vi "TEST_TankControl.vi"() -> ()   [LabVIEW 2024]
doc: "This example performs writes and reads on a serial port, as directed by the user. You can press the Write and Read buttons, and change the Read Count, while the example is running.\n\nThe parameters set for the serial port must match the parameters of the connected instrument or device. In this example, the Read Count parameter specifies the number of bytes that the serial port reads. If there were more bytes at the port than the specified number, those bytes would not be read. If there were less bytes at the port than the specified number, you would receive a timeout error.\n\nThis example expands upon the flow control options for XON and XOFF, allowing the user to choose those control characters. Also, the user can enable or disable a termination character. Some devices require a termination character in order to identify the end of command strings. Some devices send a termination character to signify the end of data to be read. This example shows how you can end the Read operation once a termination character is detected in the buffer and/or append a termination character at the end of the Write data."
uses:
  LabVIEW_InstrDriver_forLK-G3000_ver1_0_1_0/32bit/Keyence LK-G3000/Public/clusters/LKIF_FLOATVALUE.ctl
  LabVIEW_InstrDriver_forLK-G3000_ver1_0_1_0/32bit/Keyence LK-G3000/Public/enums/LKIF_FLOATRESULT.ctl
  LabVIEW_InstrDriver_forLK-G3000_ver1_0_1_0/32bit/Keyence LK-G3000/Keyence LK-G3000.lvlib
panel:
  in  "Timer ON":bool
  in  "Set Time (sec)":dbl=60.0 format="%#_13g"
  out "Time out":dbl
  out "Value 2":sgl
  out "Value":sgl
  out "Waveform Chart":dbl[][](graph)
  out "Cmd Reply":u32 format="%x"
  out "Din":i32=44 format="%x"
  out "Pump State Out":enum16{"INIT", "IDLE", "STOP", "FILL", "DRAIN"}(ring)=enum."STOP"
  out "Cmd Out":u32=56 format="%x"
  out "Message":string[](array[string])
  in  "Pump Speed":enum16{"FAST", "SLOW", "CREEP", "STOP"}(ring)=enum."CREEP"
  out "CalcData2":T1 {"LKIF_FLOATRESULT" items=["VALID", "RANGEOVER_P", "RANGEOVER_N", "WAITING"]}
  out "CalcData1":T1 {"LKIF_FLOATRESULT" items=["VALID", "RANGEOVER_P", "RANGEOVER_N", "WAITING"]}
  in  "DRAIN":bool
  in  "FILL":bool
  in  "Stop Button":bool
  # "CMD TABLE"
  # "D6(dir) D5(!en) D4(S1)  D3(S0) D2(X)  D1(X)  D0(X)   Dec\nSTOP   x       1        x      x       -     -      -        32\nINIT   1       1        1      1       -     -      -       120\nFILL   1       0        x      x       -     -      -        64\nDRAIN  0       0        x      x       -     -      -        00\n\nNONE   x       x        0      0       -     -      -        00    \nCREEP  x       x        0      1       -     -      -         8\nSLOW   x       x        1      0       -     -      -        16\nFAST   x       x        1      1       -     -      -        24"
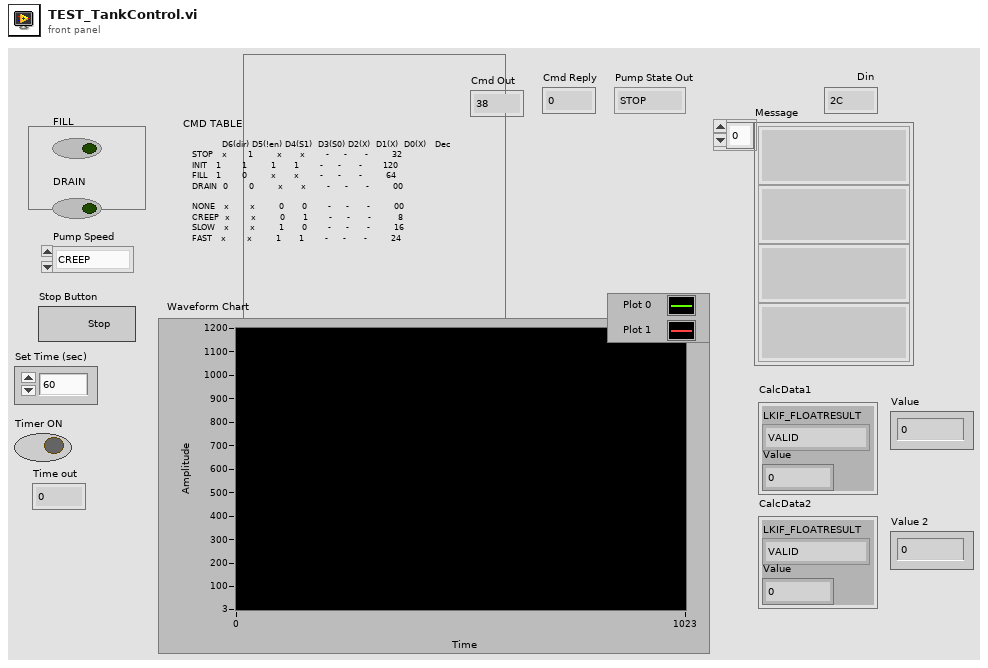
[diagram p1: front panel]
types:
  T1 = typedef "Keyence LK-G3000.lvlib/LKIF_FLOATVALUE.ctl" = cluster{"LKIF_FLOATRESULT":T2, "Value":sgl}
  T2 = typedef "Keyence LK-G3000.lvlib/LKIF_FLOATRESULT.ctl" = i32
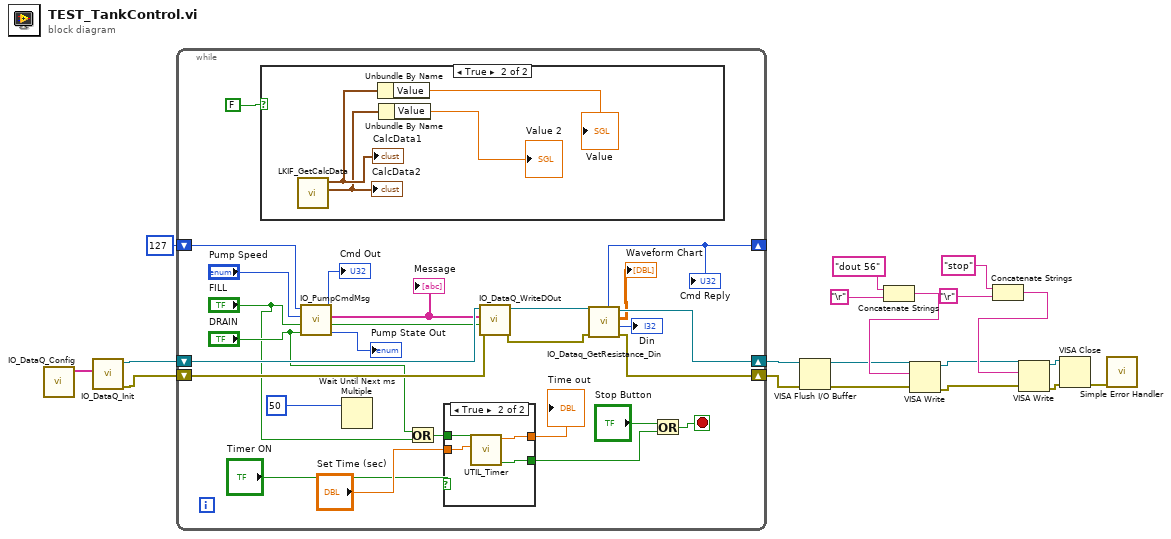
[diagram p0: block diagram]
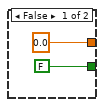
[diagram p2: hidden frame]
diagram:
  n1 = call "IO_DataQ_Config.vi"() -> ("Init Message"=w11:string[])  [unwired: 11 in]
  n2 = call "IO_DataQ_Init.vi"("Command\nList"=w11) -> ("error out"=w9:errorcluster, "VISA resource name out"=w10:refnum<visa-resource-name>)  [unwired: 8 in, 1 out]
  n3 = while {
    shift-right: [w36] -> w15
    shift-left: w10 -> [w45]
    shift-right: [w33] -> w14
    shift-left: w9 -> [w44]
    shift-right: [w30] -> _
    shift-left: u32 127 ("Cmd Out") -> [w38]
    stop <- w25 stop-if-true
    n4 = case shown="True" FALSE {
      frame False {
      }
      frame True {
        n5 = call "LKIF_GetCalcData.vi"() -> ("CalcData2"=w54:T1, "CalcData1"=w55:T1)  [unwired: 9 in, 1 out]
        "CalcData1" <- w55
        "CalcData2" <- w54
        n6 = Unbundle By Name(w55) -> ("Value"=→"Value":sgl)
        n7 = Unbundle By Name(w54) -> ("Value"=→"Value 2":sgl)
      }
    }
    n8 = call "IO_PumpCmdMsg.vi"("Drain Signal"="DRAIN", "FIll Signal"="FILL", "Pump Speed"="Pump Speed", "Cmd IN"=w38) -> ("Pump State Out"=→"Pump State Out":enum16{"INIT", "IDLE", "STOP", "FILL", "DRAIN"}, "Msg Active"=w40:bool, "Message"=w41:string[], "Cmd Out"=→"Cmd Out":u32)  [unwired: 4 in]
    "Message" <- w41
    n9 = Wait Until Next ms Multiple(millisecond multiple=50) -> ()  [unwired: 1 out]
    n10 = Or(x="DRAIN", y="FILL") -> (x .or. y?=w28:bool)
    n11 = case shown="True" "Timer ON" {
      tunnel: w28 -> [_ w51]
      tunnel: [FALSE ("Timed Out") w50] -> w23
      tunnel: [0.0 ("Numeric") w49] -> w22
      tunnel: "Set Time (sec)" -> [_ w48]
      frame False {
      }
      frame True {
        n12 = call "UTIL_Timer.vi"("Time (sec)"=w48, "Start"=w51) -> ("Timed Out"=w50:bool, "Numeric"=w49:dbl)  [unwired: 4 in, 4 out]
      }
    }
    "Time out" <- w22
    n13 = call "IO_DataQ_WriteDOut.vi"("error in (no error)"=w44, "Msg Active"=w40, "Message"=w41, "VISA Refnum in"=w45) -> ("error out"=w34:errorcluster, "VISA Refnum out"=w35:refnum<visa-resource-name>)  [unwired: 6 in]
    n14 = call "IO_Dataq_GetResistance_Din.vi"("error in (no error)"=w34, "VISA Refnum in"=w35) -> ("error out"=w33:errorcluster, "Din"=→"Din":i32, "Analog"=→"Waveform Chart":dbl[][], "VISA Refnum out"=w36:refnum<visa-resource-name>, "Cmd"=w30:u32)  [unwired: 4 in, 1 out]
    "Cmd Reply" <- w30
    n15 = Or(x="Stop Button", y=w23) -> (x .or. y?=w25:bool)
  }
  n16 = VISA Flush I/O Buffer(VISA resource name=w15, error in (no error)=w14) -> (VISA resource name out=w13:refnum<visa-resource-name>, error out=w12:errorcluster)  [unwired: 1 in]
  n17 = Concatenate Strings("dout 56", "\r") -> (w16:string)
  n18 = VISA Write(VISA resource name=w13, write buffer=w16, error in (no error)=w12) -> (VISA resource name out=w4:refnum<visa-resource-name>, error out=w3:errorcluster)  [unwired: 1 out]
  n19 = Concatenate Strings("stop", "\r") -> (w5:string)
  n20 = VISA Write(VISA resource name=w4, write buffer=w5, error in (no error)=w3) -> (VISA resource name out=w2:refnum<visa-resource-name>, error out=w1:errorcluster)  [unwired: 1 out]
  n21 = VISA Close(VISA resource name=w2, error in (no error)=w1) -> (error out=w19:errorcluster)
  n22 = call <vilib>:"Simple Error Handler.vi"("error in (no error)"=w19) -> ()  [unwired: 1 in, 8 out]
